vi "VI Server Read.vi"(1 "Action":T3=enum."Identify", 2 "Parameters":variant) -> (6 "Output":variant, 7 "Stop":bool)   [LabVIEW 2024]
uses:
  Sub Controls/Instrument Actions.ctl
  Sub Controls/Public.ctl
  Sub Controls/LV Versions Enum.ctl
  Sub Controls/User Event Command.ctl
  Sub Controls/Scan Output.ctl
panel:
  out "Measurement":dbl[](array[numeric]) format="%.2g"
  in  "Length":i32=1
  in  "Target LV Version #":T1
  in  "Start Index":i32
  in  "Indicator Label":string="Measurement"
  in  "VI Name":string="LS370 scan and read.vi"
  in  "Machine IP Address":string="PDFIGHMac.ad.magnet.fsu.edu"
  out "Title":string="VI Server Read"
  in  "Public":T2
  in  "Type":enum32{"Double Precison", "Double  Array"}(radio)
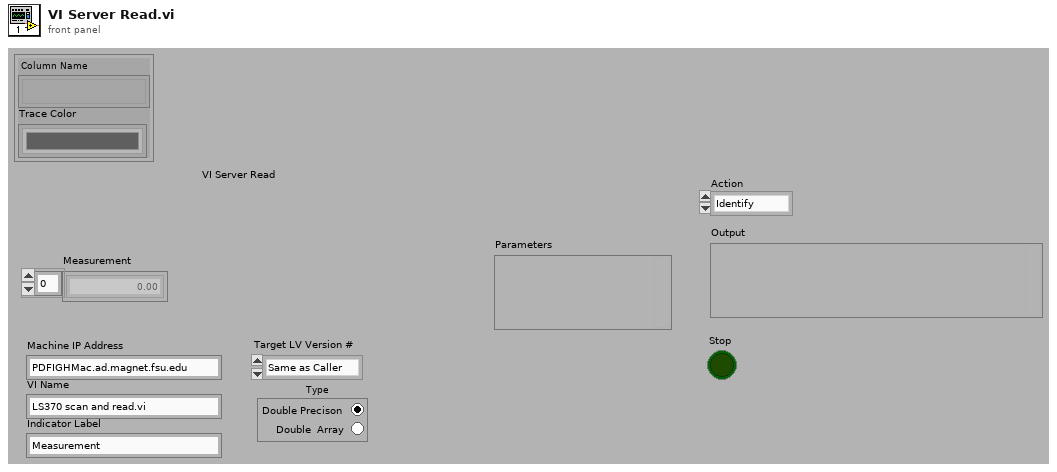
[diagram p1: front panel]
types:
  T1 = typedef "LV Versions Enum.ctl" = enum16{"Same as Caller", "8.0", "8.20", "8.5", "8.6", "9.0", "10.0", "11.0", "12.0", "13.0", "14.0", "15.0", "16.0", "17.0", "18.0", "19.0", "20.0"}
  T2 = typedef "Public.ctl" = cluster{"Column Name":string[], "Trace Color":u32[]}
  T3 = typedef "Instrument Actions.ctl" = enum16{"Scan", "Identify", "New", "Configure", "Initialize", "Test", "Read", "Close"}
  T4 = typedef "User Event Command.ctl" = enum32{"Stop Config"}
  T5 = typedef "Scan Output.ctl" = cluster{"Manufacturer":string, "Model":string, "Info":string, "Revision":string, "error out":errorcluster}
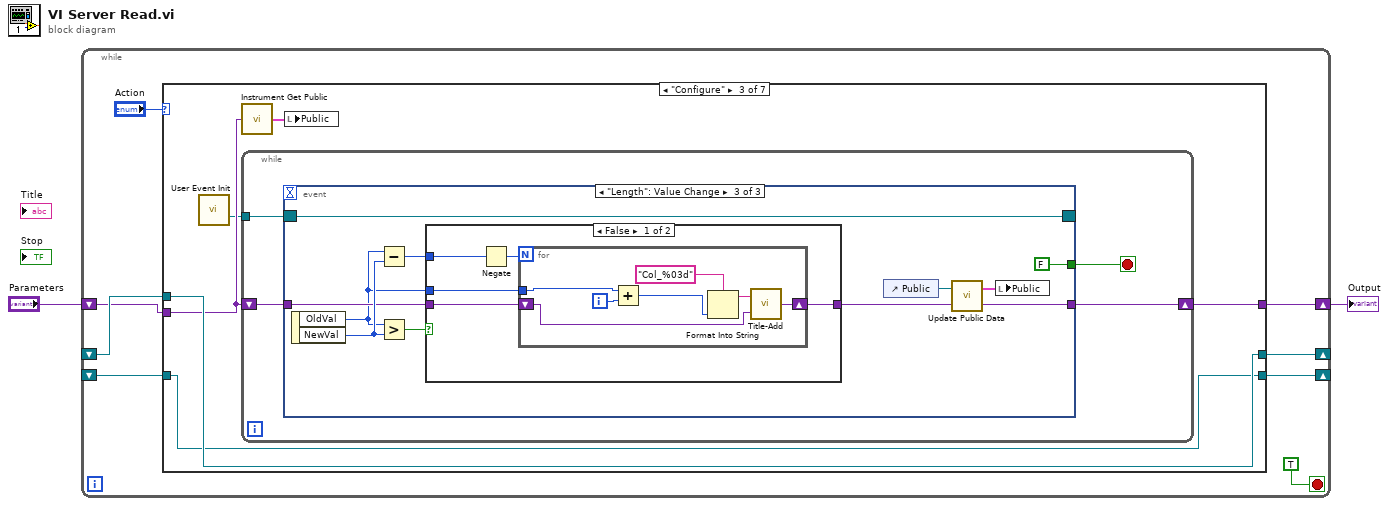
[diagram p0: block diagram]
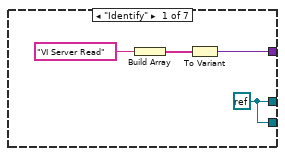
[diagram p2: hidden frame]
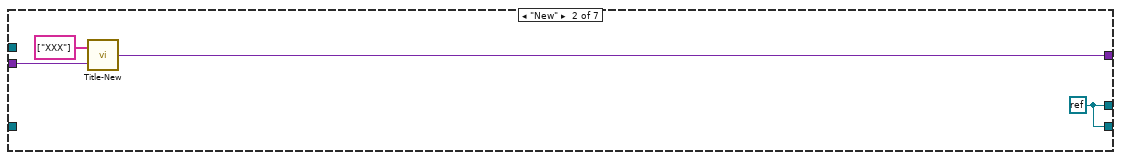
[diagram p3: hidden frame]
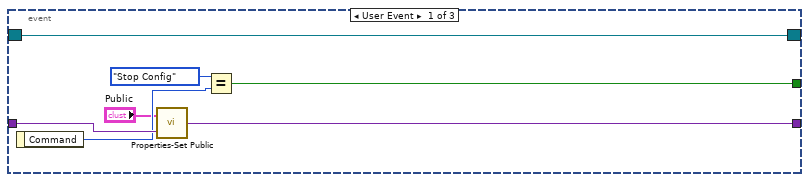
[diagram p4: hidden frame]
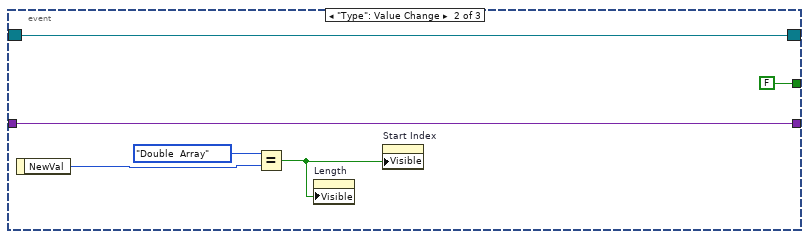
[diagram p5: hidden frame]
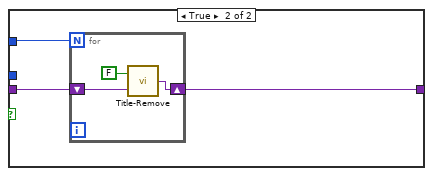
[diagram p6: hidden frame]
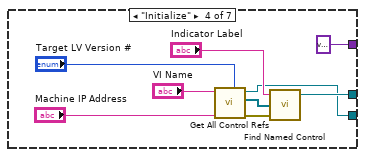
[diagram p7: hidden frame]
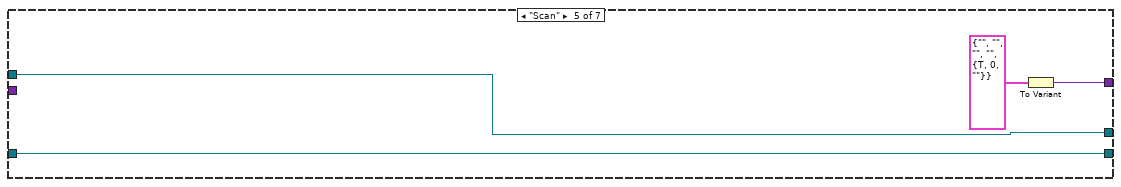
[diagram p8: hidden frame]
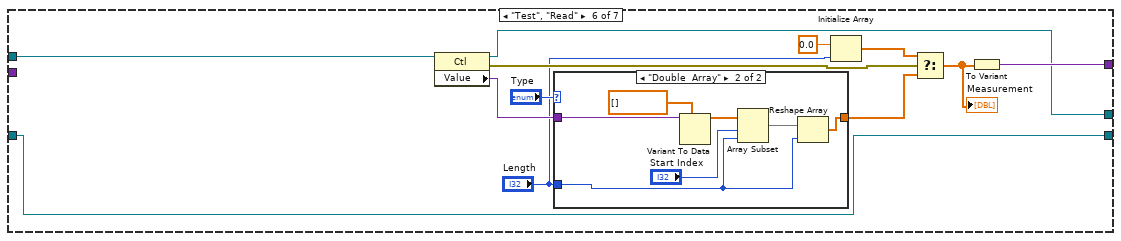
[diagram p9: hidden frame]
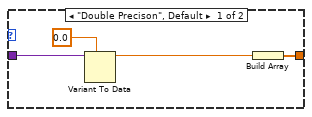
[diagram p10: hidden frame]
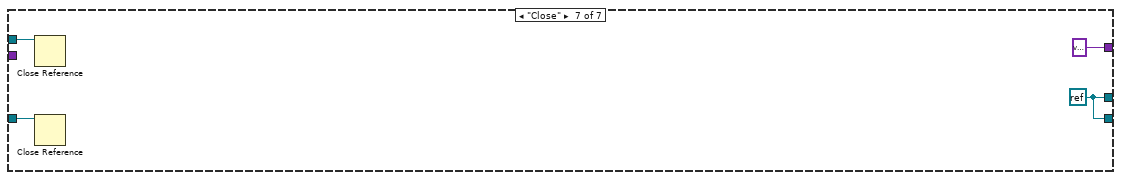
[diagram p11: hidden frame]
diagram:
  n1 = while {
    shift-right: [w9] -> _
    shift-left: _ -> [w8]
    shift-right: [w7] -> w2
    shift-left: "Parameters" -> [w6]
    shift-right: [w4] -> _
    shift-left: _ -> [w3]
    stop <- TRUE stop-if-true
    n2 = case shown="\"Configure\"" "Action" {
      tunnel: [w13 w17 w19 variant ("Variant") w82 w95 variant ("Variant")] -> w7
      tunnel: [w11 w15 w24 w74 w83 w92 w107] -> w9
      tunnel: w8 -> [_ _ w24 _ w83 w93 w110]
      tunnel: w6 -> [_ w16 w23 _ _ _ _]
      tunnel: [w11 w15 w20 w72 w80 w89 w107] -> w4
      tunnel: w3 -> [_ _ w20 _ w80 w89 w108]
      frame "Identify" {
        w11 = refnum<k0> refnum
        n3 = Build Array("VI Server Read") -> (w12:string[])
        n4 = To Variant(anything=w12) -> (Variant=w13:variant)
      }
      frame "New" {
        w15 = refnum<k0> refnum
        n5 = call "Title-New.vi"("Parameters"=w16, "Array"=string[] ["XXX"]) -> ("Instrument Prop"=w17:variant)
      }
      frame "Configure" {
        n6 = call "User Event Init.vi"() -> ("Event Registration Refnum"=w21:refnum<event-registration>)  [unwired: 14 in, 1 out]
        n7 = call "Instrument Get Public.vi"("Variant"=w23) -> ("Public"=w22:T2)
        n8 = while {
          tunnel: w21 -> [w26]
          shift-right: [w25] -> w19
          shift-left: w23 -> [w28]
          stop <- w27 stop-if-true
          n9 = event shown="[2] \"Length\": Value Change" {
            selector: w26 -> [w29 w39 w52]
            dyn-events: [w29 w39 w52] -> _
            timeout: _ -> [_ _ _]
            tunnel: [w35 w40 w44] -> w25
            tunnel: [w31 FALSE ("NewVal") FALSE ("NewVal")] -> w27
            tunnel: w28 -> [w34 w40 w47]
            event User Event {
              n10 = event-data() -> ("Command"=w33:T4)  [unwired: 1 in]
              n11 = call "Properties-Set Public.vi"("Variant"=w34, "New Public"="Public") -> ("Variant 2"=w35:variant)
              n12 = Equal?(x=User_Event_Command."Stop Config", y=w33) -> (x = y?=w31:bool)
            }
            event "Type": Value Change {
              n13 = event-data() -> ("NewVal"=w38:enum32{"Double Precison", "Double  Array"})  [unwired: 1 in]
              n14 = Equal?(x=enum32{"Double Precison", "Double  Array"}."Double  Array", y=w38) -> (x = y?=w36:bool)
              n15 = property on="Length" class="DigNum (strict)"("Visible"=w36) -> ()  [unwired: 2 in, 2 out]
              n16 = property on="Start Index" class="DigNum (strict)"("Visible"=w36) -> ()  [unwired: 2 in, 2 out]
            }
            event "Length": Value Change {
              n17 = event-data() -> ("OldVal"=w46:i32, "NewVal"=w49:i32)  [unwired: 1 in]
              n18 = Subtract(x=w46, y=w49) -> (x-y=w48:i32)
              n19 = Greater?(x=w46, y=w49) -> (0:w50:bool)
              n20 = case shown="False" w50 {
                tunnel: w48 -> [w57 w67]
                tunnel: w47 -> [w56 w66]
                tunnel: [w55 w65] -> w45
                tunnel: w46 -> [w53 _]
                frame False {
                  n21 = Negate(x=w57) -> (-x=w54:i32)
                  n22 = for {
                    N: w54 -> [_]
                    shift-right: [w64] -> w55
                    shift-left: w56 -> [w63]
                    tunnel: w53 -> [w58]
                    i -> [w59]
                    n23 = Add(x=w58, y=w59) -> (x+y=w60:i32)
                    n24 = Format Into String(format string="Col_%03d", w60) -> (resulting string=w62:string)  [unwired: 2 in, 1 out]
                    n25 = call "Title-Add.vi"("Parameters"=w63, "String"=w62) -> ("Variant"=w64:variant)
                  }
                }
                frame True {
                  n26 = for {
                    N: w67 -> [_]
                    shift-right: [w69] -> w65
                    shift-left: w66 -> [w70]
                    n27 = call "Title-Remove.vi"("Parameters"=w70, "Remove First"=FALSE) -> ("Variant"=w69:variant)
                  }
                }
              }
              n28 = control-ref of="Public"() -> (w42:refnum<vi>)
              n29 = call "Update Public Data.vi"("Variant In"=w45, "Public 2"=w42) -> ("Variant Out"=w44:variant, "Public"=w43:T2)
              n30 = local write "Public"(w43) -> ()
            }
          }
        }
        n31 = local write "Public"(w22) -> ()
      }
      frame "Initialize" {
        n32 = call "Get All Control Refs.vi"("VI Name"="VI Name", "Machine Name"="Machine IP Address", "Target LV Version #"="Target LV Version #") -> ("VI Refnum"=w72:refnum<vi>, "All Controls"=w78:refnum<vi>[], "error out"=w77:errorcluster)  [unwired: 3 in]
        n33 = call "Find Named Control.vi"("error in"=w77, "All Controls"=w78, "Control Name"="Indicator Label") -> ("Ctl Refnum"=w74:refnum<vi>)  [unwired: 2 out]
      }
      frame "Scan" {
        n34 = To Variant(anything=T5 {"Manufacturer"="", "Model"="", "Info"="", "Revision"="", "error out"={"status"=TRUE, "code"=0, "source"=""}} ("Scan Output")) -> (Variant=w82:variant)
      }
      frame "Test", "Read" {
        n35 = property class="Ctl"(reference=w93) -> (reference out=w92:refnum<vi>, error out=w91:errorcluster, "Value"=w90:variant)  [unwired: 1 in]
        n36 = case shown="\"Double  Array\"" "Type" {
          tunnel: w90 -> [w99 w105]
          tunnel: [w96 w100] -> w85
          tunnel: "Length" -> [_ w102]
          frame "Double Precison", Default {
            n37 = Variant To Data(type=0.0, Variant=w99) -> (data=w97:dbl)  [unwired: 1 in, 1 out]
            n38 = Build Array(w97) -> (w96:dbl[])
          }
          frame "Double  Array" {
            n39 = Variant To Data(type=dbl[] [], Variant=w105) -> (data=w104:dbl[])  [unwired: 1 in, 1 out]
            n40 = Array Subset(array=w104, index="Start Index", length=w102) -> (w101:dbl[])
            n41 = Reshape Array(w101, w102) -> (w100:dbl[])
          }
        }
        n42 = Initialize Array(0.0, "Length") -> (w87:dbl[])
        n43 = Select(t=w87, s=w91, f=w85) -> (s? t:f=w84:dbl[])
        "Measurement" <- w84
        n44 = To Variant(anything=w84) -> (Variant=w95:variant)
      }
      frame "Close" {
        w107 = refnum<k0> refnum
        n45 = Close Reference(reference=w110) -> ()  [unwired: 1 in, 1 out]
        n46 = Close Reference(reference=w108) -> ()  [unwired: 1 in, 1 out]
      }
    }
  }
  "Output" <- w2
